vi "PrepareDeviceListForDisplay.vi"(1 "DAQ Device List":string[][](array[string])) -> (0 "PreparedDeviceListForDisplay":string[](array[string]))   [LabVIEW 2017]
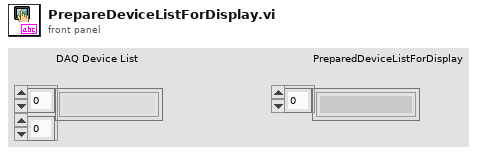
[diagram p1: front panel]
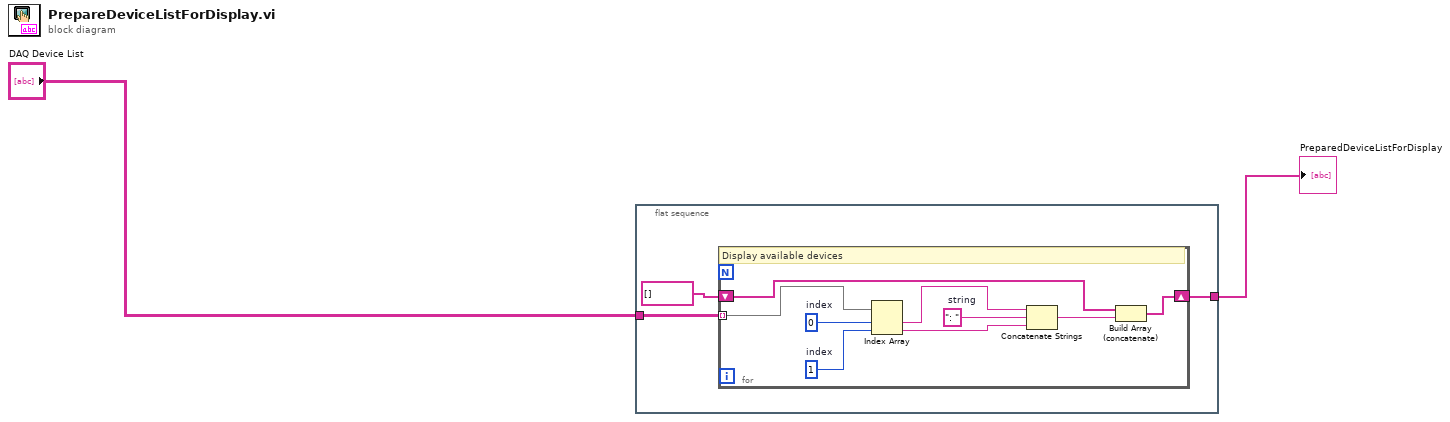
[diagram p0: block diagram]
diagram:
  n1 = flat-sequence {
    tunnel: [w4] -> w1
    tunnel: "DAQ Device List" -> [w3]
    frame #0 {
      n2 = for {
        tunnel: w3 -> [w14] mode=indexing
        shift-right: [w11] -> w4
        shift-left: string[] [] -> [w12]
        w8 = ": "  # string
        w10 = 1  # index
        w13 = 0  # index
        # "Display available devices"
        n3 = Index Array(array=w14, index #1=w13, index #2=w10) -> (element #1=w9:string, element #2=w7:string)
        n4 = Concatenate Strings(w9, w8, w7) -> (w6:string)
        n5 = Build Array (concatenate)(w12, w6) -> (w11:string[])
      }
    }
  }
  "PreparedDeviceListForDisplay" <- w1
